vi "ChromaProtectionStatus.vi"(8 "error in (no error)":errorcluster, 11 "ChromaAcLoad in":refnum<class "ChromaAcLoad.lvclass">) -> (0 "error out":errorcluster, 3 "ChromaAcLoad out":refnum<class "ChromaAcLoad.lvclass">)   [LabVIEW 2018, in "AcPwrPlugins.lvlib" / "ChromaAcLoad.lvclass"]
uses:
  ChromaAcLoad.lvclass
  C:/Users/ico/Documents/Projects/NistPluggableModules/AcPwr/AcPwrPlugins/AcPwrBaseClass/AcPwrBase.lvclass
  AcPwrBaseClass/AcPwrBase.lvclass/AcPwrBase.ctl
  AcPwrBaseClass/Accessors/Read BaseMeasurements.vi
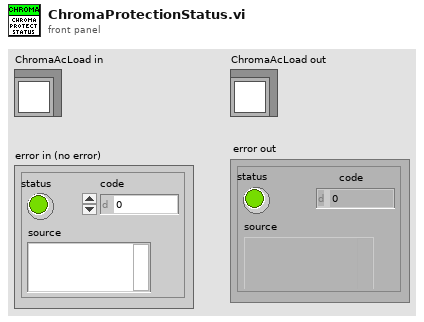
[diagram p1: front panel]
types:
  T1 = typedef "AcPwrPlugins.lvlib/AcPwrBase.lvclass/BaseMeasurements.ctl" = cluster{"Handle":string, "Name":string, "Enabled":bool, "Measurement Value":dbl, "btnMeasFetch":bool, "Chroma Hold Peak Current Measurement":bool, "Chroma Measurement Type":T2, "Chroma Protection Status String":string, "NHRDC Fetch Method":i32, "NHRDC Fetch Time (s)":sgl, "NHRDC Measurement Type":i32, "NHRGridSim Measurement Type ":enum16{"Average Current", "Max Current", "Min Current", "Average Voltage", "Max Voltage", "Min Voltage", "Average True Power", "Max True Power", "Min True Power", "Average Apparent Power", "Max Apparent Power", "Min Apparent Power", "Power Factor", "Crest Factor"}, "NHRGridSim Phase ":i32, "PPS Measurement Type ":enum16{"Voltage RMS L-N", "Voltage RMS L-L", "Frequency", "Current RMS", "Current Peak", "Crest Factor", "Power Factor", "Power VA", "Real Power"}, "PPS Channel Name":enum16{"A", "B", "C"}}[]
  T2 = typedef "AcPwrPlugins.lvlib/ChromaAcLoad.lvclass/MeasurementType.ctl" = enum16{"Voltage (Vrms or V)", "Current (Arms or A)", "Power (W)", "Peak Voltage (V)", "Peak Current (A)", "Peak Power (W)", "Frequency (Hz)", "Resistance (Ohms)", "Voltage Overshoot (V)", "Positive Peak Current (A)", "Voltage Undershoot (V)", "Negative Peak Current (A)", "Apparent Power (VA)", "Reacitive Power (VAR)", "Voltage THD", "Power Factor", "Current's Crest Factor"}
  T3 = cluster{"Handle":string, "Name":string, "Enabled":bool, "Measurement Value":dbl, "btnMeasFetch":bool, "Chroma Hold Peak Current Measurement":bool, "Chroma Measurement Type":T2, "Chroma Protection Status String":string, "NHRDC Fetch Method":i32, "NHRDC Fetch Time (s)":sgl, "NHRDC Measurement Type":i32, "NHRGridSim Measurement Type ":enum16{"Average Current", "Max Current", "Min Current", "Average Voltage", "Max Voltage", "Min Voltage", "Average True Power", "Max True Power", "Min True Power", "Average Apparent Power", "Max Apparent Power", "Min Apparent Power", "Power Factor", "Crest Factor"}, "NHRGridSim Phase ":i32, "PPS Measurement Type ":enum16{"Voltage RMS L-N", "Voltage RMS L-L", "Frequency", "Current RMS", "Current Peak", "Crest Factor", "Power Factor", "Power VA", "Real Power"}, "PPS Channel Name":enum16{"A", "B", "C"}}
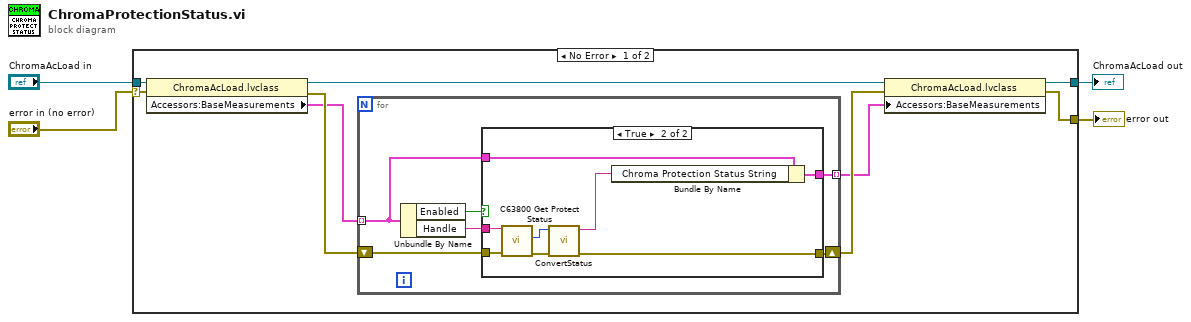
[diagram p0: block diagram]
diagram:
  n1 = case shown="No Error" "error in (no error)" {
    selector: "error in (no error)" -> [w10 w30]
    tunnel: [w8 w31] -> w4
    tunnel: [w7 w30] -> w3
    tunnel: "ChromaAcLoad in" -> [w11 w31]
    frame No Error {
      n2 = property class="ChromaAcLoad.lvclass"(reference=w11, error in=w10) -> (reference out=w9:refnum<class "ChromaAcLoad.lvclass">, error out=w13:errorcluster, "Accessors:BaseMeasurements"=w12:T1)
      n3 = for {
        tunnel: w12 -> [w15] mode=indexing
        shift-right: [w18] -> w6
        shift-left: w13 -> [w19]
        tunnel: [w14] -> w5 mode=indexing
        n4 = Unbundle By Name(w15) -> ("Enabled"=w16:bool, "Handle"=w17:string)
        n5 = case shown="True" w16 {
          tunnel: w19 -> [w21 w29]
          tunnel: [w21 w23] -> w18
          tunnel: w17 -> [_ w28]
          tunnel: w15 -> [w20 w27]
          tunnel: [w20 w26] -> w14
          frame False {
          }
          frame True {
            n6 = call <instrlib>:"C63800 Get Protect Status.vi"("error in (no error)"=w29, "Instrument Handle"=w28) -> ("error out"=w25:errorcluster, "Protect Status"=w24:i32)  [unwired: 7 in, 1 out]
            n7 = call "ConvertStatus.vi"("Error In"=w25, "Protect Status"=w24) -> ("Error Out"=w23:errorcluster, "Numeric Indicator"=w22:string)  [unwired: 8 in]
            n8 = Bundle By Name(cluster=w27, "Chroma Protection Status String"=w22) -> (w26:T3)
          }
        }
      }
      n9 = property class="ChromaAcLoad.lvclass"(reference=w9, error in=w6, "Accessors:BaseMeasurements"=w5) -> (reference out=w8:refnum<class "ChromaAcLoad.lvclass">, error out=w7:errorcluster)
    }
    frame Error {
    }
  }
  "ChromaAcLoad out" <- w4
  "error out" <- w3
